vi "FPGA实物信号仿真.vi"() -> ()   [LabVIEW 2012]
uses:
  <vilib>/Analysis/NI_AALBase.lvlib
  <vilib>/Analysis/3filter.llb/Butterworth Filter (DBL).vi
  P3060NEW/_SubVI/dll/P3060.dll
panel:
  out "entire buffer [read all]":dbl[](array[numeric]) caption="全部缓冲区[读取全部]" format="%0.2f"
  in  "打开串口按钮":bool caption="空白按钮"
  out "Elements in Queue":i32(slide) caption="队列中的元素" scale=0.0..200.0 scale format="%0.0f"
  in  "Enqueue Element":bool caption="元素入队列"
  out "时域/频域切换":bool
  in  "设置按钮":bool
  in  "板卡单次传输点数":u32=8192
  out "error out":errorcluster caption="错误输出"
  in  "槽位号":i16=6
  in  "取消按钮":bool
  in  "FPGA-Bit文件路径":path
  in  "加载程序":bool caption="确定按钮"
  out "波形图":i32[](graph)
  in  "read":bool caption="显示采集卡数据"
  in  "板卡LED控制":bool
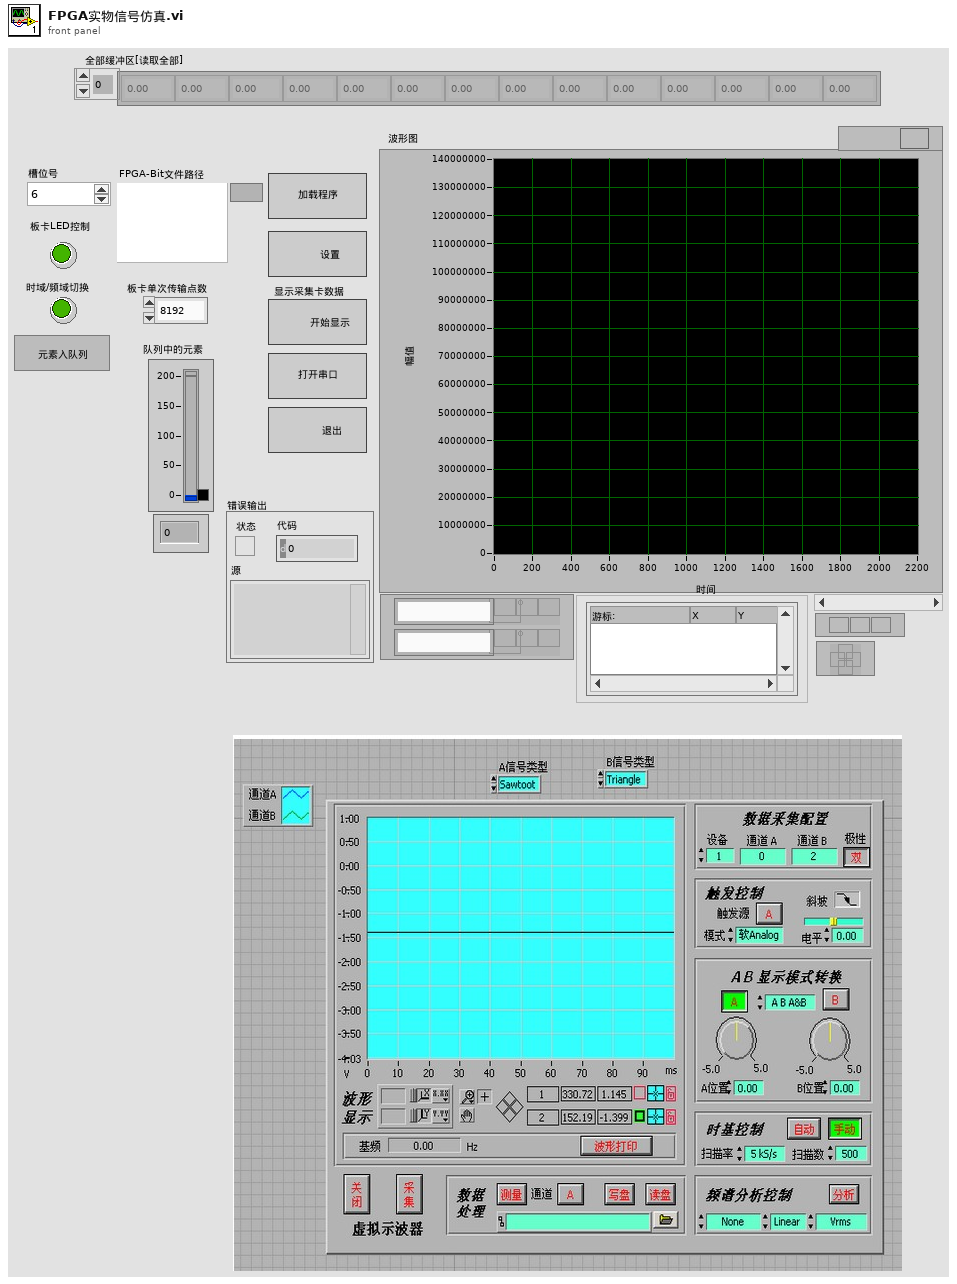
[diagram p1: front panel]
types:
  T1 = enum16{"empty", "write", "read oldest (queue)", "read newest (stack)", "read all"}
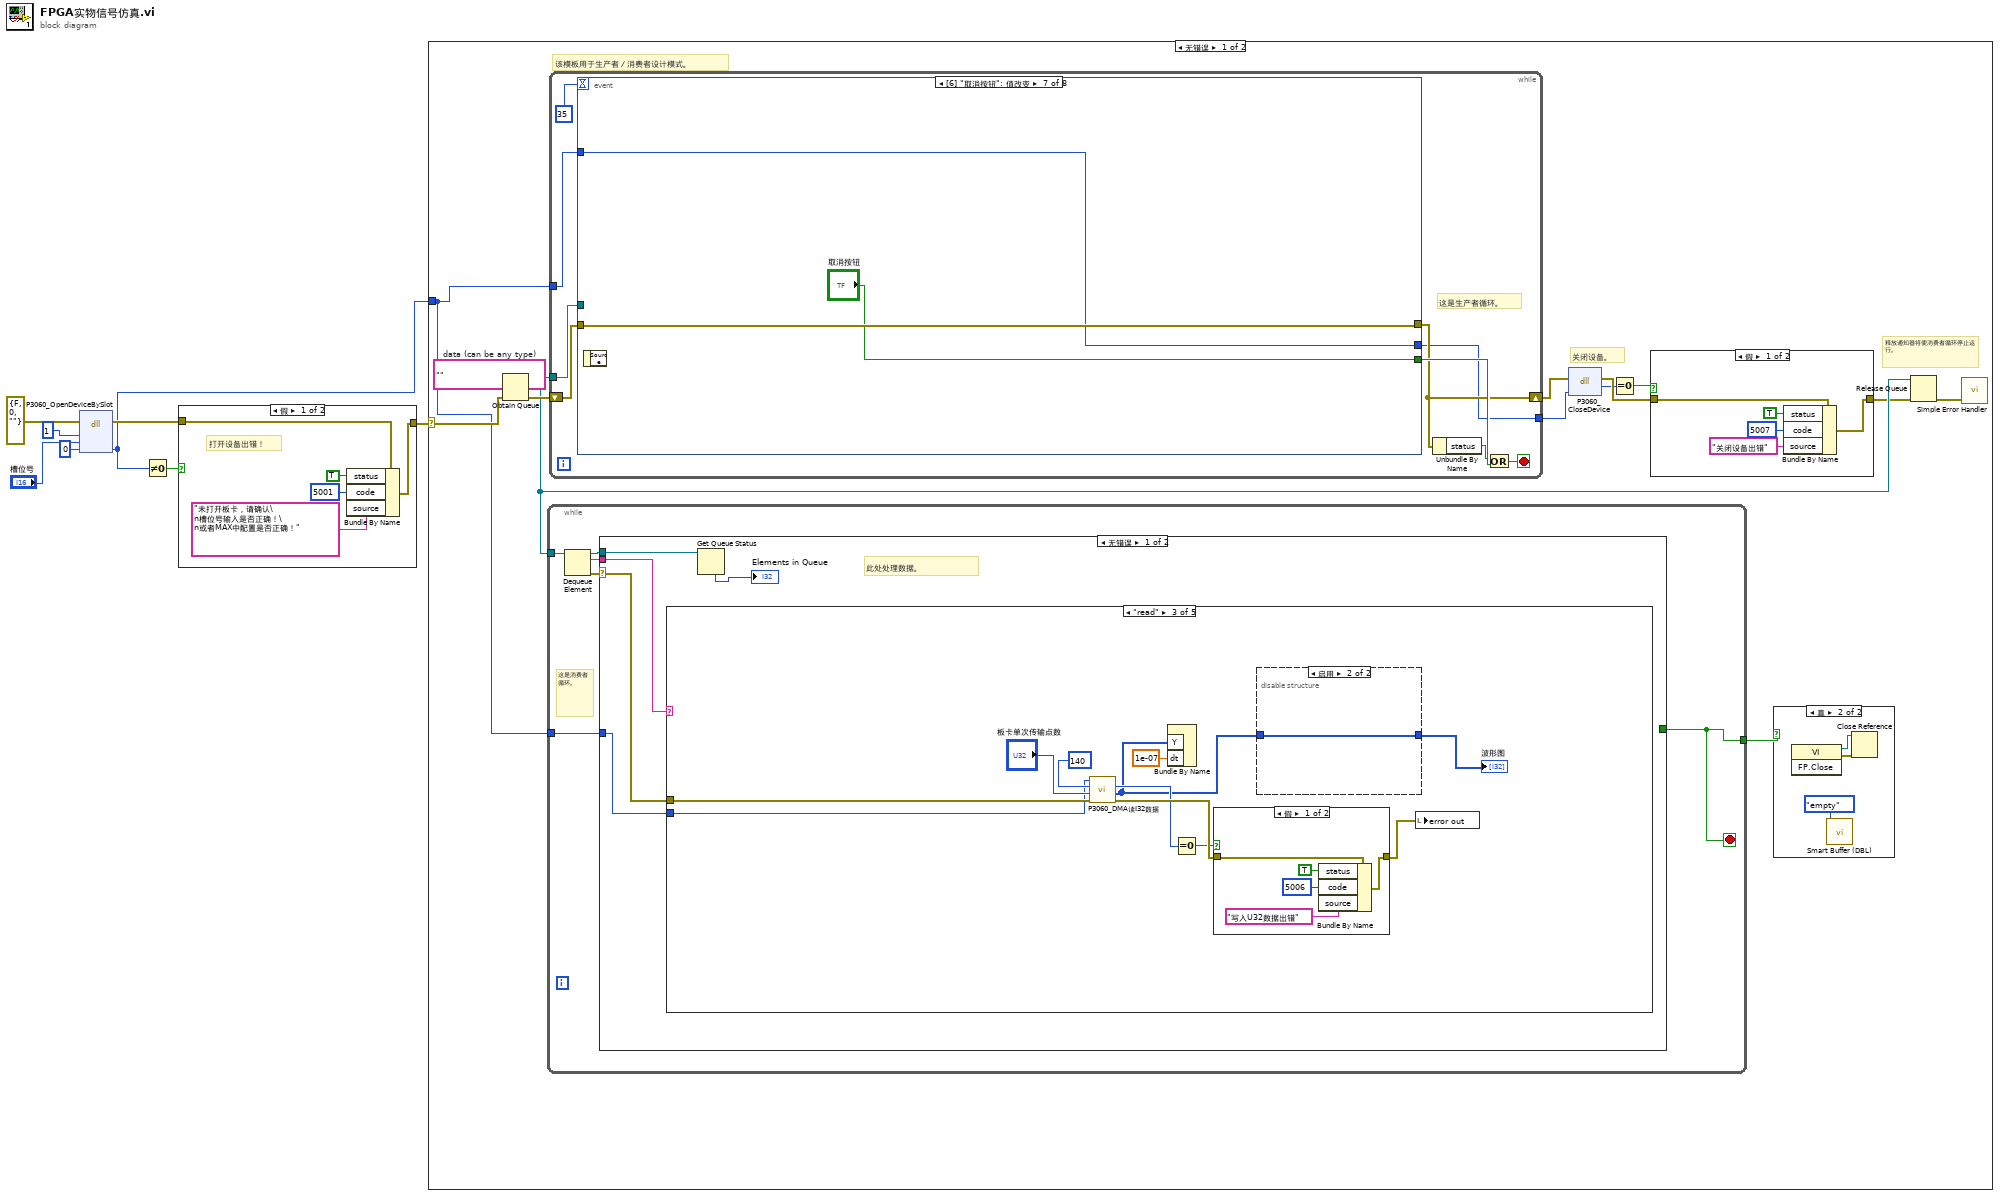
[diagram p0: block diagram]
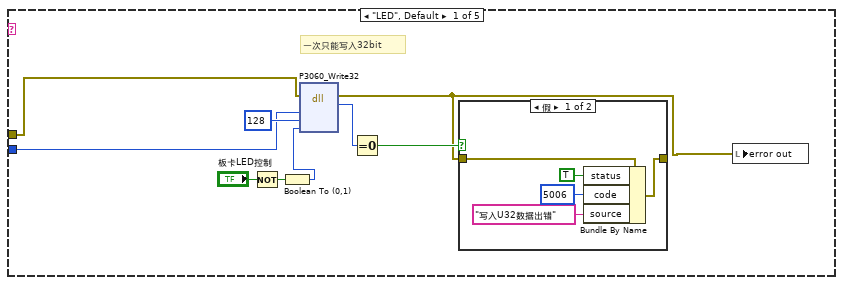
[diagram p4: hidden frame]
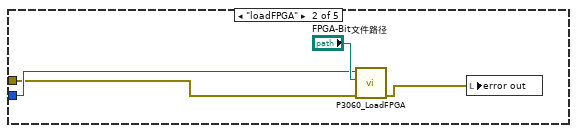
[diagram p6: hidden frame]
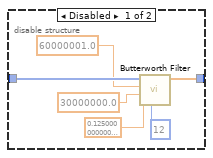
[diagram p7: hidden frame]
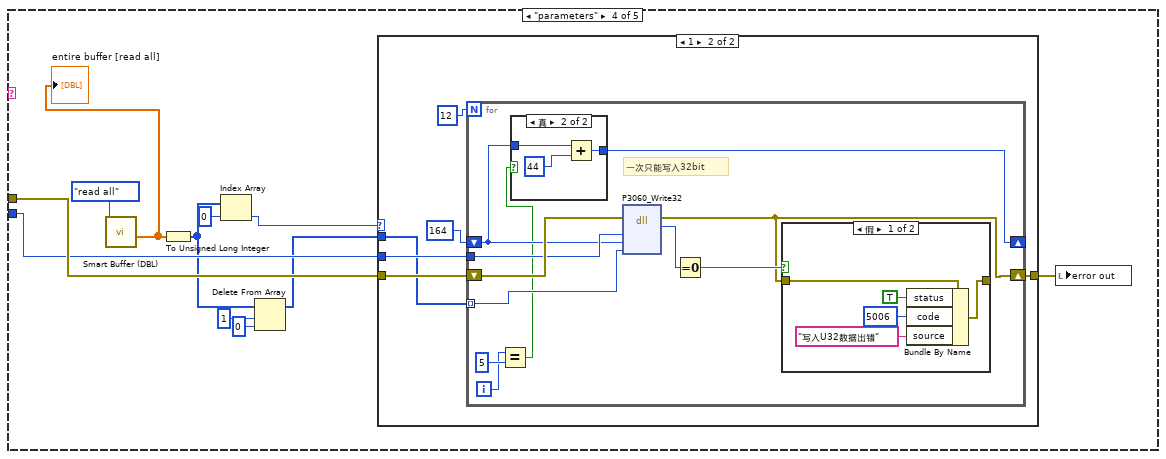
[diagram p9: hidden frame]
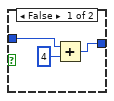
[diagram p11: hidden frame]
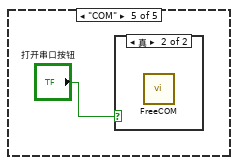
[diagram p13: hidden frame]
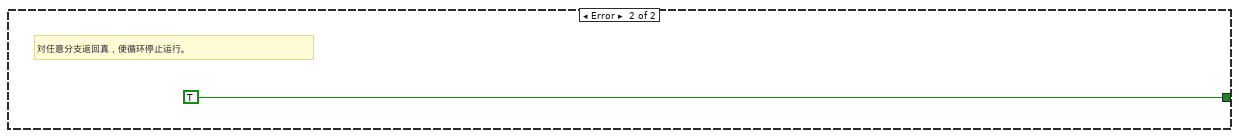
[diagram p15: hidden frame]
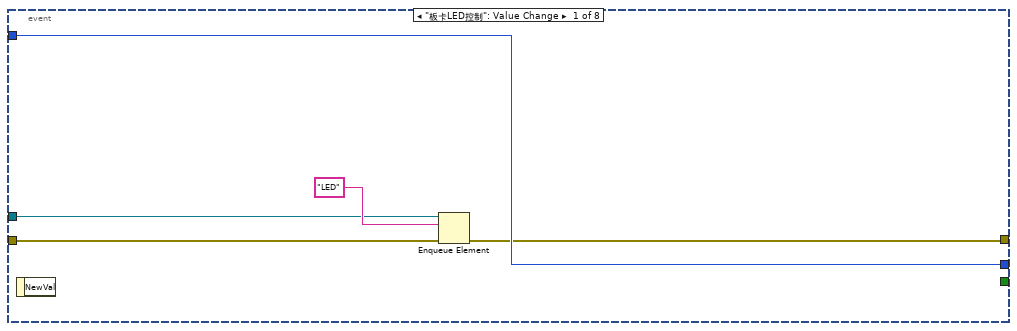
[diagram p16: hidden frame]
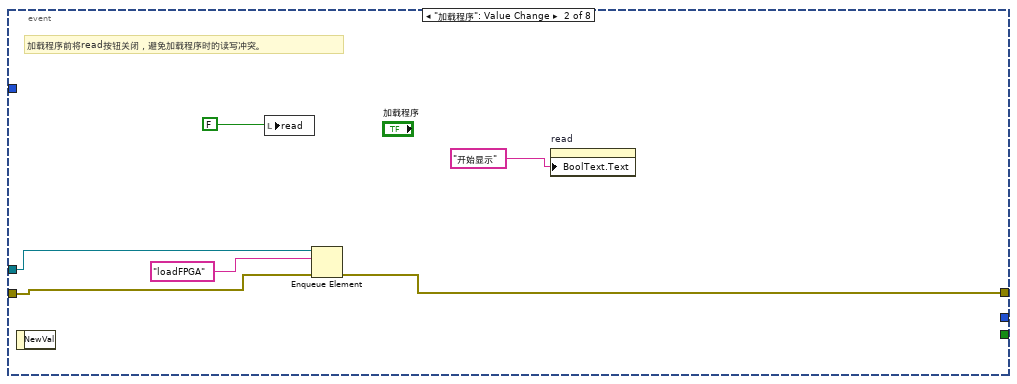
[diagram p17: hidden frame]
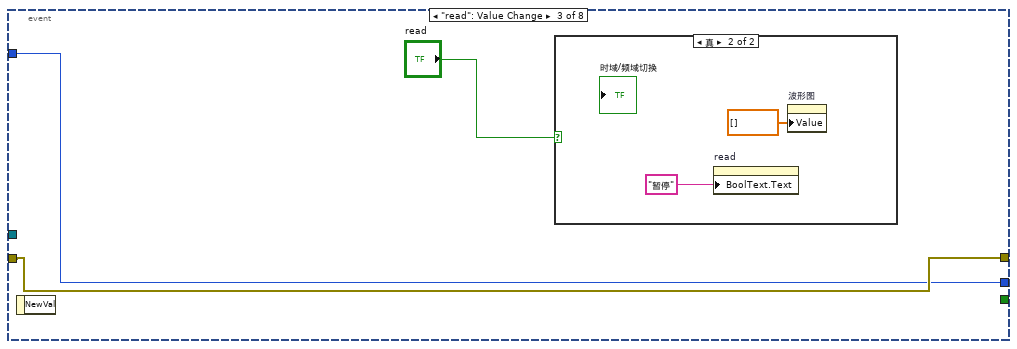
[diagram p18: hidden frame]
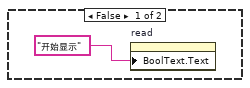
[diagram p19: hidden frame]
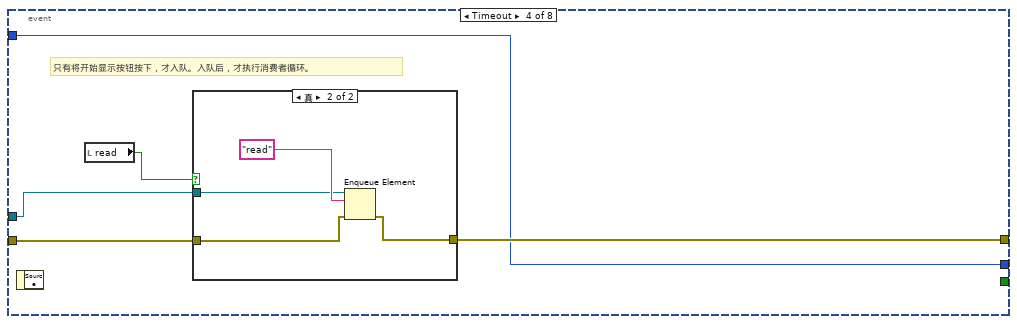
[diagram p20: hidden frame]
diagram:
  n1 = dll-call lib="C:/PLC_simulation/2014.3.13PLC_NEW/PLC_NEW/P3060NEW/_SubVI/dll/P3060.dll" fn="P3060_OpenDeviceBySlot"(error in=errorcluster {"status"=FALSE, "code"=0, "source"=""} ("error IO"), "Classis"=i16 1, "槽位号"="槽位号", "设备句柄"=0) -> (error out=w8:errorcluster, "设备句柄"=w1:i32)  [unwired: 5 in, 1 out]
  n2 = Not Equal To 0?(x=w1) -> (x != 0?=w5:bool)
  n3 = case shown="假" w5 {
    tunnel: w8 -> [w13 w14]
    tunnel: [w9 w14] -> w2
    frame False {
      # "打开设备出错！"
      n4 = Bundle By Name(cluster=w13, "status"=TRUE, "code"=5001, "source"="未打开板卡，请确认\n槽位号输入是否正确！\n或者MAX中配置是否正确！") -> (w9:errorcluster)
    }
    frame True {
      # "打开设备成功！"
    }
  }
  n5 = case shown="无错误" w2 {
    selector: w2 -> [w19 w208]
    tunnel: w1 -> [w15 _]
    frame No Error {
      w26 = ""  # data (can be any type)
      # "关闭设备。"
      # "释放通知器将使消费者循环停止运行。"
      # "该模板用于生产者／消费者设计模式。"
      n6 = Obtain Queue(element data type=w26, error in (no error)=w19) -> (queue out=w25:refnum<queue>, error out=w27:errorcluster)  [unwired: 3 in, 1 out]
      n7 = while {
        tunnel: w25 -> [w42]
        tunnel: [w38] -> w24
        tunnel: w15 -> [w39]
        stop <- w38 stop-if-true
        # "这是消费者循环。"
        n8 = Dequeue Element(queue=w42) -> (queue out=w37:refnum<queue>, element=w40:string, error out=w41:errorcluster)  [unwired: 2 in, 1 out]
        n9 = case shown="无错误" w41 {
          selector: w41 -> [w47 _]
          tunnel: w40 -> [w45 _]
          tunnel: [_ TRUE] -> w38
          tunnel: w39 -> [w46 _]
          tunnel: w37 -> [w44 _]
          frame No Error {
            # "此处处理数据。"
            n10 = case shown="\"read\"" w45 {
              tunnel: w47 -> [w50 w64 w72 w99 _]
              tunnel: w46 -> [w49 w65 w71 w98 _]
              frame "LED", Default {
                # "一次只能写入32bit"
                n11 = Not(x="板卡LED控制") -> (.not. x?=w52:bool)
                n12 = Boolean To (0,1)(Boolean=w52) -> (0, 1=w53:i16)
                n13 = dll-call lib="C:/PLC_simulation/2014.3.13PLC_NEW/PLC_NEW/P3060NEW/_SubVI/dll/P3060.dll" fn="P3060_Write32"(error in=w50, "hDev"=w49, "Offset"=u32 128, "data"=w53) -> (error out=w48:errorcluster, "return"=w56:i32)  [unwired: 5 in, 1 out]
                n14 = Equal To 0?(x=w56) -> (x = 0?=w55:bool)
                n15 = case shown="假" w55 {
                  tunnel: [w60 w62] -> _
                  tunnel: w48 -> [w61 w62]
                  frame False {
                    n16 = Bundle By Name(cluster=w61, "status"=TRUE, "code"=5006, "source"="写入U32数据出错") -> (w60:errorcluster)
                  }
                  frame True {
                  }
                }
                n17 = local write "error out"(w48) -> ()
              }
              frame "loadFPGA" {
                n18 = call "P3060_LoadFPGA.vi"("错误输入"=w64, "Bit文件路径"="FPGA-Bit文件路径", "句柄输入"=w65) -> ("错误输出"=w63:errorcluster)  [unwired: 6 in, 2 out]
                n19 = local write "error out"(w63) -> ()
              }
              frame "read" {
                n20 = call "P3060_DMA读I32数据.vi"("错误输入"=w72, "数据长度"="板卡单次传输点数", "偏移地址"=u32 140, "句柄输入"=w71) -> ("错误输出"=w77:errorcluster, "读I32数据"=w68:i32[], "返回值"=w74:i32)  [unwired: 4 in, 1 out]
                n21 = Bundle By Name ("创建波形")("Y"=w68, "dt"=1e-07) -> ()  [unwired: 1 in, 1 out]
                n22 = Equal To 0?(x=w74) -> (x = 0?=w73:bool)
                n23 = case shown="假" w73 {
                  tunnel: [w88 w90] -> w70
                  tunnel: w77 -> [w89 w90]
                  frame False {
                    n24 = Bundle By Name(cluster=w89, "status"=TRUE, "code"=5006, "source"="写入U32数据出错") -> (w88:errorcluster)
                  }
                  frame True {
                  }
                }
                n25 = disable-structure shown="启用" {
                  disable-tunnel: w68 -> [w83 w84]
                  disable-tunnel: [w78 w84] -> w67
                  frame Disabled {
                    n26 = call-poly <vilib>:"Butterworth Filter.vi"("order"=12, "low cutoff freq: fl"=0.12500000000000006, "high cutoff freq: fh"=30000000.0, "sampling freq: fs"=60000001.0, "X"=w83) -> ("Filtered X"=w78:dbl[])  [unwired: 3 in, 1 out]
                  }
                  frame Enabled {
                  }
                }
                "波形图" <- w67
                n27 = local write "error out"(w70) -> ()
              }
              frame "parameters" {
                n28 = call "Smart Buffer (DBL).vi"("mode"=T1."read all") -> ("entire buffer [read all]"=w97:dbl[])  [unwired: 5 in, 5 out]
                "entire buffer [read all]" <- w97
                n29 = To Unsigned Long Integer(number=w97) -> (unsigned 32bit integer=w94:u32[])
                n30 = Index Array(array=w94, index=0 ("索引")) -> (element=w95:u32)
                n31 = Delete From Array(array=w94, length=1 ("长度"), index=0 ("索引")) -> (array with subset deleted=w91:u32[])  [unwired: 1 out]
                n32 = case shown="1" w95 {
                  tunnel: [w102 w108] -> w100
                  tunnel: w99 -> [w102 w107]
                  tunnel: w98 -> [_ w106]
                  tunnel: w91 -> [_ w104]
                  frame 0, Default {
                  }
                  frame 1 {
                    n33 = for {
                      N: 12 -> [_]
                      tunnel: w106 -> [w115]
                      shift-right: [w117] -> w108
                      shift-left: w107 -> [w116]
                      shift-right: [w109] -> _
                      shift-left: u32 164 ("Offset") -> [w114]
                      tunnel: w104 -> [w113] mode=indexing
                      i -> [w110]
                      # "一次只能写入32bit"
                      n34 = Equal?(x=w110, y=5) -> (x = y?=w111:bool)
                      n35 = case shown="真" w111 {
                        tunnel: w114 -> [w120 w124]
                        tunnel: [w121 w123] -> w109
                        frame False {
                          n36 = Add(x=w120, y=4 ("x")) -> (x+y=w121:u32)
                        }
                        frame True {
                          n37 = Add(x=w124, y=44 ("x")) -> (x+y=w123:u32)
                        }
                      }
                      n38 = dll-call lib="C:/PLC_simulation/2014.3.13PLC_NEW/PLC_NEW/P3060NEW/_SubVI/dll/P3060.dll" fn="P3060_Write32"(error in=w116, "hDev"=w115, "Offset"=w114, "data"=w113) -> (error out=w117:errorcluster, "return"=w119:i32)  [unwired: 5 in, 1 out]
                      n39 = Equal To 0?(x=w119) -> (x = 0?=w118:bool)
                      n40 = case shown="假" w118 {
                        tunnel: [w129 w131] -> _
                        tunnel: w117 -> [w130 w131]
                        frame False {
                          n41 = Bundle By Name(cluster=w130, "status"=TRUE, "code"=5006, "source"="写入U32数据出错") -> (w129:errorcluster)
                        }
                        frame True {
                        }
                      }
                    }
                  }
                }
                n42 = local write "error out"(w100) -> ()
              }
              frame "COM" {
                n43 = case shown="真" "打开串口按钮" {
                  frame False {
                  }
                  frame True {
                    n44 = call "FreeCOM.vi"() -> ()  [unwired: 12 in]
                  }
                }
              }
            }
            n45 = Get Queue Status(queue=w44) -> (# elements in queue=→"Elements in Queue":i32)  [unwired: 2 in, 7 out]
          }
          frame Error {
            # "对任意分支返回真，使循环停止运行。"
          }
        }
      }
      n46 = while {
        shift-right: [w138] -> w18
        shift-left: w27 -> [w141]
        tunnel: w25 -> [w142]
        tunnel: w15 -> [w135]
        tunnel: [w134] -> w16
        stop <- w139 stop-if-true
        # "这是生产者循环。"
        n47 = event shown="[6] \"取消按钮\": 值改变" {
          selector: _ -> [_ _ _ _ _ _ _ _]
          dyn-events: _ -> [_ _ _ _ _ _ _ _]
          timeout: 35 -> [_ _ _ _ _ _ _ _]
          tunnel: w142 -> [w144 w150 _ w164 w172 w199 _ w207]
          tunnel: w141 -> [w145 w152 w155 w163 w171 w198 w203 w206]
          tunnel: [w143 w151 w155 w162 w170 w197 w203 w205] -> w138
          tunnel: [_ _ _ _ _ _ "取消按钮" _] -> w140
          tunnel: w135 -> [w146 _ w154 w161 _ _ w201 _]
          tunnel: [w146 _ w154 w161 _ _ w201 _] -> w134
          event "板卡LED控制": Value Change {
            n48 = event-data() -> ()  [unwired: 1 in, 1 out]
            n49 = Enqueue Element(queue=w144, element="LED", error in (no error)=w145) -> (error out=w143:errorcluster)  [unwired: 1 in, 2 out]
          }
          event "加载程序": Value Change {
            # "加载程序前将read按钮关闭，避免加载程序时的读写冲突。"
            n50 = event-data() -> ()  [unwired: 1 in, 1 out]
            n51 = local write "read"(FALSE) -> ()
            n52 = Enqueue Element(queue=w150, element="loadFPGA", error in (no error)=w152) -> (error out=w151:errorcluster)  [unwired: 1 in, 2 out]
            n53 = property on="read" class="Bool (严格)"("BoolText.Text"="开始显示") -> ()  [unwired: 2 in, 2 out]
          }
          event "read": Value Change {
            n54 = event-data() -> ()  [unwired: 1 in, 1 out]
            n55 = case shown="真" "read" {
              frame False {
                n56 = property on="read" class="Bool (严格)"("BoolText.Text"="开始显示") -> ()  [unwired: 2 in, 2 out]
              }
              frame True {
                n57 = property on="read" class="Bool (严格)"("BoolText.Text"="暂停") -> ()  [unwired: 2 in, 2 out]
                n58 = property on="波形图" class="WFGraph (严格)"("Value"=dbl[] [] ("波形图")) -> ()  [unwired: 2 in, 2 out]
              }
            }
          }
          event Timeout {
            # "只有将开始显示按钮按下，才入队。入队后，才执行消费者循环。"
            n59 = event-data() -> ()  [unwired: 1 in, 1 out]
            n60 = local read "read"() -> (w160:bool)
            n61 = case shown="真" w160 {
              tunnel: w164 -> [_ w168]
              tunnel: w163 -> [w165 w167]
              tunnel: [w165 w166] -> w162
              frame False {
              }
              frame True {
                n62 = Enqueue Element(queue=w168, element="read", error in (no error)=w167) -> (error out=w166:errorcluster)  [unwired: 1 in, 2 out]
              }
            }
          }
          event "设置按钮": Value Change {
            n63 = event-data() -> ()  [unwired: 1 in, 1 out]
            n64 = case shown="真" "设置按钮" {
              tunnel: w172 -> [_ w176]
              tunnel: w171 -> [_ w175]
              tunnel: [_ w174] -> w170
              frame False {
              }
              frame True {
                n65 = local write "设置按钮"(FALSE ("布尔")) -> ()
                n66 = local write "read"(FALSE) -> ()
                n67 = flat-sequence {
                  tunnel: w176 -> [w194]
                  tunnel: w175 -> [w193]
                  tunnel: [w192] -> w174
                  frame #0 {
                    n68 = property class="VI"("FP:RunTransparently"=TRUE ("前面板窗口:以透明方式运行VI"), "FP:Transparency"=u8 100 ("前面板窗口:透明度")) -> ()  [unwired: 2 in, 2 out]
                  }
                  frame #1 {
                    n69 = Current VI's Path() -> (path=w181:path)
                    n70 = Strip Path(path=w181) -> (stripped path=w191:path)  [unwired: 1 out]
                    n71 = Build Path(base path=w191, name or relative path="参数配置.vi" ("名称或相对路径")) -> (appended path=w190:path)
                    n72 = Open VI Reference(vi path=w190) -> (vi reference=w189:refnum<vi>, error out=w188:errorcluster)  [unwired: 5 in]
                    n73 = property class="VI"(reference=w189, error in=w188, "Front Panel.Open"=TRUE ("前面板窗口:打开")) -> (reference out=w186:refnum<vi>, error out=w185:errorcluster)
                    n74 = invoke class="VI" method="Run VI"(reference=w186, error in=w185, "Wait until done"=TRUE ("结束前等待"), "Auto Dispose Ref"=TRUE ("自动销毁引用")) -> ()  [unwired: 1 in, 5 out]
                  }
                  frame #2 {
                    n75 = property class="VI"("FP:RunTransparently"=FALSE ("前面板窗口:以透明方式运行VI")) -> ()  [unwired: 2 in, 2 out]
                    n76 = Enqueue Element(queue=w194, element="parameters", error in (no error)=w193) -> (error out=w192:errorcluster)  [unwired: 1 in, 2 out]
                  }
                }
              }
            }
          }
          event "打开串口按钮": Value Change {
            n77 = event-data() -> ()  [unwired: 1 in, 1 out]
            n78 = Enqueue Element(queue=w199, element="COM", error in (no error)=w198) -> (error out=w197:errorcluster)  [unwired: 1 in, 2 out]
          }
          event "取消按钮": Value Change {
            n79 = event-data() -> ()  [unwired: 1 in, 1 out]
          }
          event "Enqueue Element": Value Change {
            # "此处生成数据。"
            n80 = event-data() -> ()  [unwired: 1 in, 1 out]
            n81 = Enqueue Element(queue=w207, element="element", error in (no error)=w206) -> (error out=w205:errorcluster)  [unwired: 1 in, 2 out]
          }
        }
        n82 = Unbundle By Name(w138) -> ("status"=w137:bool)
        n83 = Or(x=w137, y=w140) -> (x .or. y?=w139:bool)
      }
      n84 = dll-call lib="C:/PLC_simulation/2014.3.13PLC_NEW/PLC_NEW/P3060NEW/_SubVI/dll/P3060.dll" fn="P3060_CloseDevice"(error in=w18, "hDev"=w16) -> (error out=w23:errorcluster, "hDevOut"=w21:i32)  [unwired: 3 in, 1 out]
      n85 = Equal To 0?(x=w21) -> (x = 0?=w22:bool)
      n86 = case shown="假" w22 {
        tunnel: [w31 w33] -> w17
        tunnel: w23 -> [w32 w33]
        frame False {
          n87 = Bundle By Name(cluster=w32, "status"=TRUE, "code"=5007, "source"="关闭设备出错") -> (w31:errorcluster)
        }
        frame True {
        }
      }
      n88 = case shown="真" w24 {
        frame False {
        }
        frame True {
          n89 = invoke class="VI" method="FP.Close"() -> (reference out=w35:refnum<vi>, error out=w36:errorcluster)  [unwired: 3 in, 1 out]
          n90 = call "Smart Buffer (DBL).vi"("mode"=T1."empty") -> ()  [unwired: 5 in, 6 out]
          n91 = Close Reference(reference=w35, error in (no error)=w36) -> ()  [unwired: 1 out]
        }
      }
      n92 = Release Queue(queue=w25, error in (no error)=w17) -> (error out=w20:errorcluster)  [unwired: 1 in, 2 out]
      n93 = call <vilib>:"Simple Error Handler.vi"("error in (no error)"=w20) -> ()  [unwired: 4 in, 5 out]
    }
    frame Error {
      # "此处使用顺序结构而没有采用错误输出相连接这种更为优雅的方式，是因为后者会导致弹出两个错误提示窗口，即便删除前边的错误处理器，这个VI在遇到设备不能打开的时候也不会自己关闭。"
      n94 = flat-sequence {
        tunnel: w208 -> [w209]
        frame #0 {
          n95 = call <vilib>:"Simple Error Handler.vi"("error in (no error)"=w209) -> ()  [unwired: 4 in, 5 out]
        }
        frame #1 {
          n96 = invoke class="VI" method="FP.Close"() -> (reference out=w210:refnum<vi>, error out=w211:errorcluster)  [unwired: 3 in, 1 out]
          n97 = Close Reference(reference=w210, error in (no error)=w211) -> ()  [unwired: 1 out]
        }
      }
      "error out" <- w208
    }
  }
